vi "read.vi"(6 "call chain index (1)":i32=1, 7 "vi ref (caller)":refnum<vi>, 8 "error in (no error)":errorcluster) -> (0 "error out":errorcluster, 2 "module id":i32, 3 "status control id":i32)   [LabVIEW 2024, in "status manager.lvlib"]
uses:
  status manager.lvlib
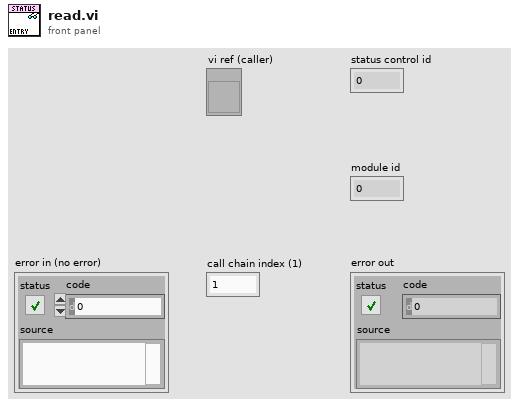
[diagram p1: front panel]
types:
  T1 = typedef "status manager.lvlib/entry type.ctl" = cluster{"status control id":i32, "module id":i32}
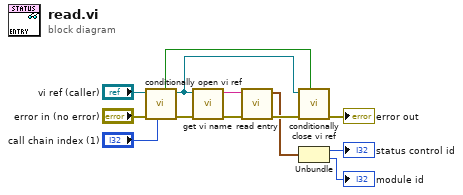
[diagram p0: block diagram]
diagram:
  n1 = call "conditionally open vi ref.vi"("call chain index (1)"="call chain index (1)", "error in (no error)"="error in (no error)", "vi ref in"="vi ref (caller)") -> ("error out"=w13:errorcluster, "vi ref out"=w10:refnum<vi>, "new ref?"=w9:bool)  [unwired: 6 in]
  n2 = call "get vi name.vi"("error in (no error)"=w13, "vi ref"=w10) -> ("error out"=w6:errorcluster, "vi name"=w4:string)  [unwired: 8 in]
  n3 = call "read entry.vi"("error in (no error)"=w6, "id"=w4) -> ("error out"=w5:errorcluster, "entry"=w3:T1)  [unwired: 8 in]
  n4 = call "conditionally close vi ref.vi"("new ref?"=w9, "error in (no error)"=w5, "vi ref"=w10) -> ("error out"=→"error out":errorcluster)  [unwired: 8 in]
  n5 = Unbundle(w3) -> ("status control id"=→"status control id":i32, "module id"=→"module id":i32)
